vi "OpenImaq.vi"() -> (0 "error out":errorcluster, 1 "IMAQ Session Out":refnum<k11>)   [LabVIEW 2010]
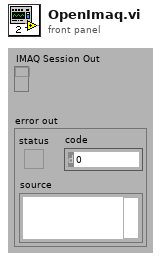
[diagram p1: front panel]
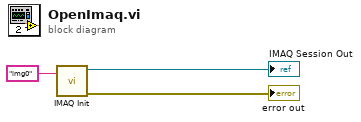
[diagram p0: block diagram]
diagram:
  n1 = call <vilib>:"IMAQ Init.vi"("Interface Name"="img0") -> ("error out"=→"error out":errorcluster, "IMAQ Session Out"=→"IMAQ Session Out":refnum<k11>)  [unwired: 9 in]
